vi "NI DOCO DEMO.vi"() -> ()   [LabVIEW 2018]
uses:
  <vilib>/DAQmx/write.llb/DAQmx Write (Digital Wfm 1Chan NSamp).vi
  <vilib>/DAQmx/write.llb/DAQmx Write (Analog Wfm 1Chan NSamp).vi
  <vilib>/DAQmx/create/channels.llb/DAQmx Create Channel (AO-Voltage-Basic).vi
  <vilib>/DAQmx/configure/timing.llb/DAQmx Timing (Sample Clock).vi
  <vilib>/DAQmx/create/channels.llb/DAQmx Create Channel (DO-Digital Output).vi
  <vilib>/Waveform/DWDTOps.llb/DWDT Boolean Array to Digital.vi
  <vilib>/Waveform/WDTOps.llb/WDT Append Waveforms DBL.vi
  <vilib>/DAQmx/miscellaneous.llb/DAQmx Fill In Error Info.vi
  <vilib>/Waveform/DWDTOps.llb/DWDT Uncompress Digital.vi
  <vilib>/Waveform/DWDTOps.llb/DWDT Append Digital Samples.vi
  <vilib>/measure/NI_MABase.lvlib
panel:
  out "Numeric":u32
  in  "Enum":enum16{"A A", "A B", "B B", "B A"}(ring)
  in  "stop 2":bool
  out "Mixed Signal Graph":T1(graph)
  in  "stop":bool
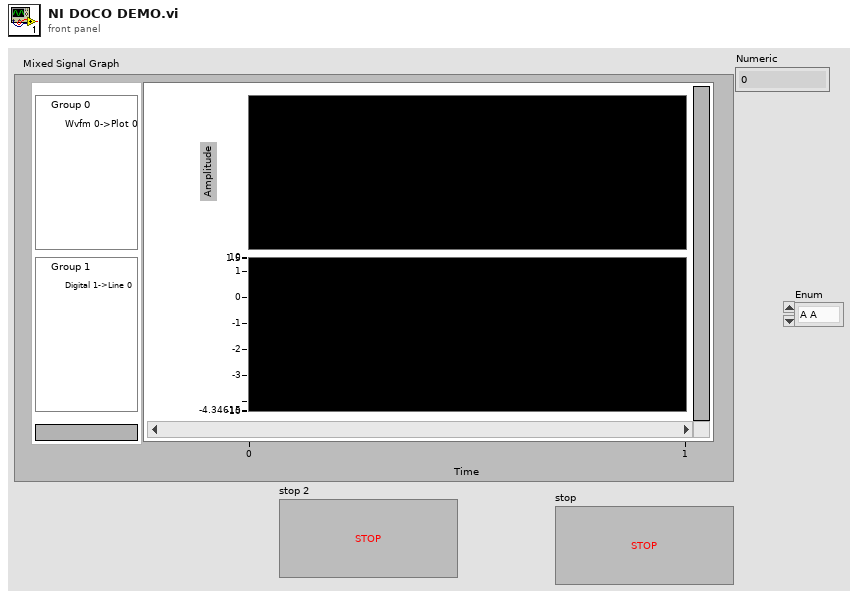
[diagram p1: front panel]
types:
  T1 = cluster{"signal out":waveform(dbl), "digital waveform":digitalwaveform}
  T2 = cluster{"waveform out":waveform(dbl), "output waveform":digitalwaveform}
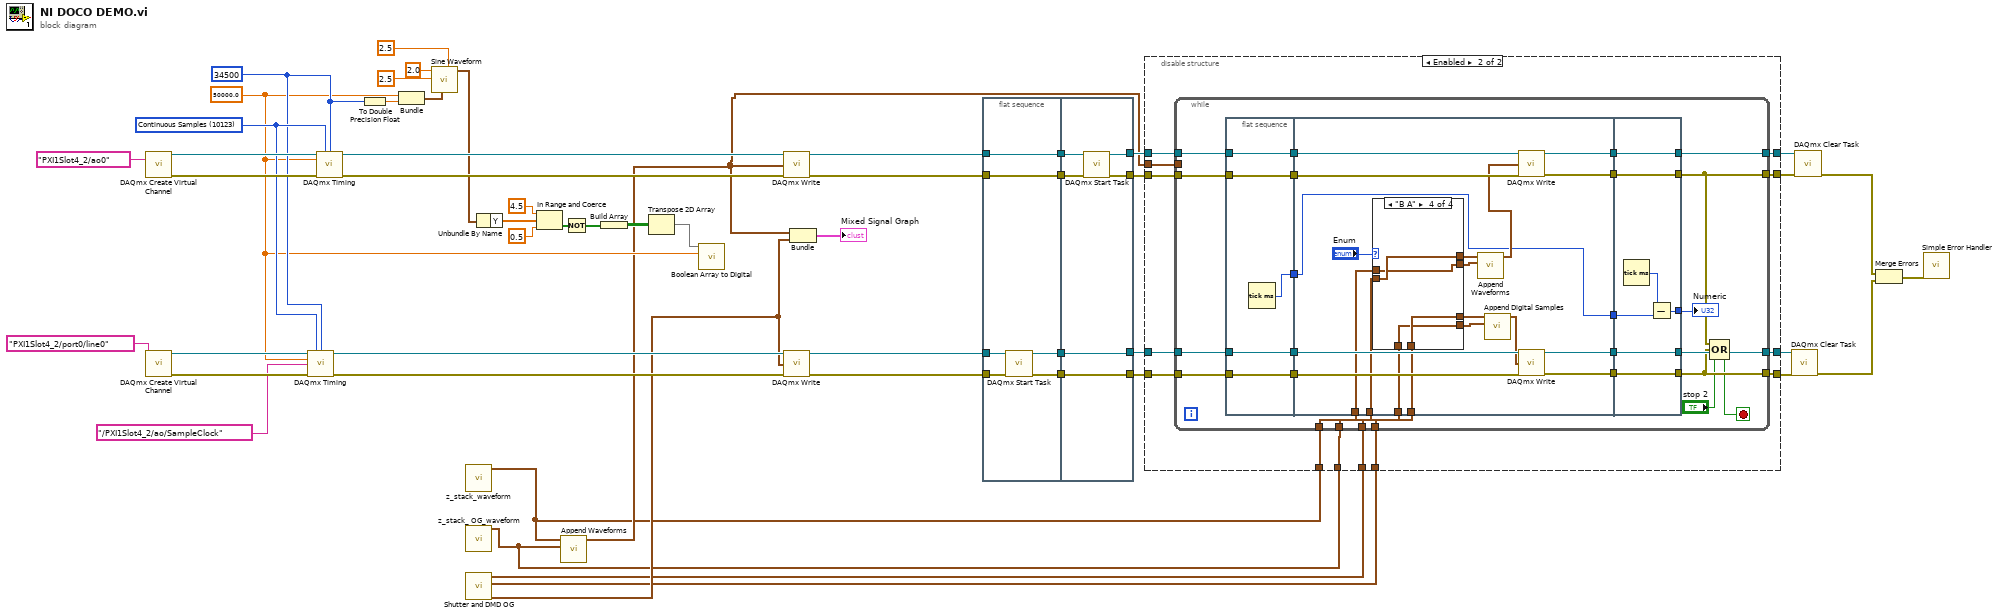
[diagram p0: block diagram]
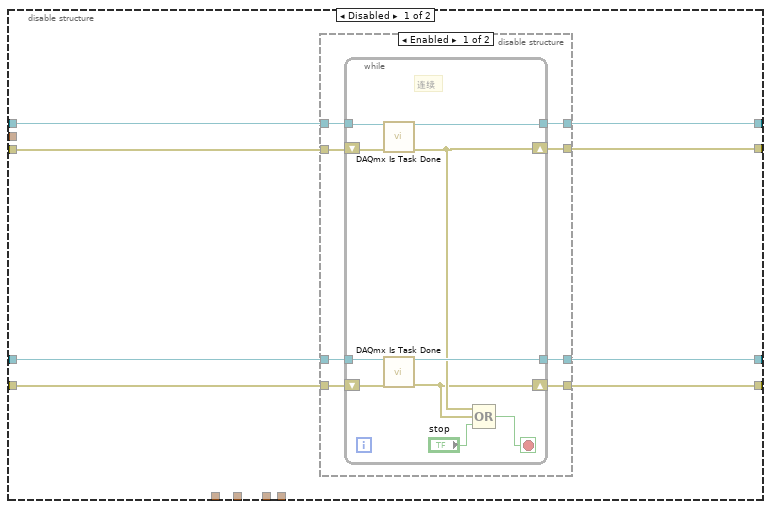
[diagram p2: hidden frame]
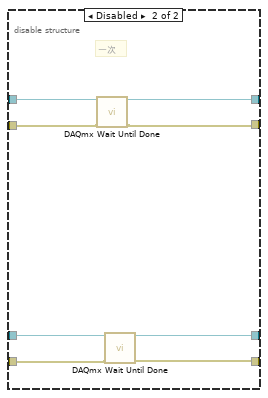
[diagram p3: hidden frame]
diagram:
  w42 = 34500 ("samples per channel")
  w47 = 10123 items=["Finite Samples"=10178, "Continuous Samples"=10123, "Hardware Timed Single Point"=12522] ("sample mode")
  w14 = 50000.0 ("rate")
  n1 = call-poly <vilib>:"DAQmx Create Virtual Channel.vi"("physical channels"=tag "PXI1Slot4_2/ao0") -> ("task out"=w52:refnum<k21>, "error out"=w51:errorcluster)  [unwired: 13 in]
  n2 = call-poly <vilib>:"DAQmx Create Virtual Channel.vi"("lines"=tag "PXI1Slot4_2/port0/line0") -> ("task out"=w48:refnum<k21>, "error out"=w49:errorcluster)  [unwired: 13 in]
  n3 = call-poly <vilib>:"DAQmx Timing.vi"("task/channels in"=w48, "sample mode"=w47, "samples per channel"=w42, "rate"=w14, "source"=tag "/PXI1Slot4_2/ao/SampleClock", "error in"=w49) -> ("task out"=w12:refnum<k21>, "error out"=w9:errorcluster)  [unwired: 8 in]
  n4 = call-poly <vilib>:"DAQmx Timing.vi"("task/channels in"=w52, "sample mode"=w47, "samples per channel"=w42, "rate"=w14, "error in"=w51) -> ("task out"=w45:refnum<k21>, "error out"=w44:errorcluster)  [unwired: 9 in]
  n5 = To Double Precision Float(number=w42) -> (double precision float=w43:dbl)
  n6 = Bundle("rate"=w14, w43) -> (w41:cluster{"rate":dbl, dbl})  [unwired: 1 in]
  n7 = call <vilib>:"Sine Waveform.vi"("offset"=2.5, "sampling info"=w41, "amplitude"=2.5, "frequency"=2.0) -> ("signal out"=w8:waveform(dbl))  [unwired: 6 in, 1 out]
  n8 = call "z_stack_waveform.vi"() -> ("waveform out"=w4:waveform(dbl))  [unwired: 9 in, 2 out]
  n9 = call "z_stack_ OG_waveform.vi"() -> ("waveform out"=w3:waveform(dbl))  [unwired: 15 in, 4 out]
  n10 = call "Shutter and DMD OG.vi"() -> ("output waveform"=w5:digitalwaveform, "output waveform 2"=w1:digitalwaveform, "output waveform1"=w2:digitalwaveform)  [unwired: 8 in]
  n11 = Unbundle By Name(w8) -> ("Y"=w20:dbl[])
  n12 = In Range and Coerce(upper limit=4.5 ("offset"), x=w20, lower limit=0.5 ("offset")) -> (In Range?=w17:bool[])  [unwired: 1 out]
  n13 = call-poly <vilib>:"Append Waveforms.vi"("waveform B"=w3, "waveform A"=w4) -> ("waveform out"=w6:waveform(dbl))  [unwired: 8 in, 1 out]
  n14 = Not(x=w17) -> (.not. x?=w16:bool[])
  n15 = Build Array(w16) -> (w15:bool[][])
  n16 = Transpose 2D Array(2D array=w15) -> (transposed array=w13:bool[][])
  n17 = call-poly <vilib>:"Boolean Array to Digital.vi"("sample rate"=w14, "boolean array"=w13) -> ()  [unwired: 8 in, 2 out]
  n18 = call-poly <vilib>:"DAQmx Write.vi"("task/channels in"=w45, "data"=w6, "error in"=w44) -> ("task out"=w37:refnum<k21>, "error out"=w33:errorcluster)  [unwired: 10 in, 1 out]
  n19 = call-poly <vilib>:"DAQmx Write.vi"("task/channels in"=w12, "data"=w5, "error in"=w9) -> ("task out"=w11:refnum<k21>, "error out"=w10:errorcluster)  [unwired: 10 in, 1 out]
  n20 = Bundle("waveform out"=w6, "output waveform"=w5) -> (→"Mixed Signal Graph":T2)  [unwired: 1 in]
  n21 = flat-sequence {
    tunnel: w37 -> [w59]
    tunnel: w11 -> [w58]
    tunnel: w10 -> [w57]
    tunnel: [w59] -> w36
    tunnel: [w56] -> w35
    tunnel: [w55] -> w34
    tunnel: w33 -> [w54]
    tunnel: [w54] -> w32
    tunnel: w36 -> [w63]
    tunnel: [w65] -> w29
    tunnel: w35 -> [w65]
    tunnel: [w64] -> w28
    tunnel: w34 -> [w64]
    tunnel: [w62] -> w31
    tunnel: w32 -> [w61]
    tunnel: [w60] -> w30
    frame #0 {
      n22 = call <vilib>:"DAQmx Start Task.vi"("task/channels in"=w58, "error in"=w57) -> ("task out"=w56:refnum<k21>, "error out"=w55:errorcluster)  [unwired: 12 in]
    }
    frame #1 {
      n23 = call <vilib>:"DAQmx Start Task.vi"("task/channels in"=w63, "error in"=w61) -> ("task out"=w62:refnum<k21>, "error out"=w60:errorcluster)  [unwired: 12 in]
    }
  }
  n24 = disable-structure shown="Enabled" {
    disable-tunnel: w31 -> [w73 w112]
    disable-tunnel: w30 -> [w72 w111]
    disable-tunnel: w29 -> [w71 w110]
    disable-tunnel: w28 -> [w70 w109]
    disable-tunnel: [w69 w107] -> w27
    disable-tunnel: [w68 w108] -> w26
    disable-tunnel: [w67 w106] -> w25
    disable-tunnel: [w66 w105] -> w24
    disable-tunnel: w6 -> [_ w104]
    disable-tunnel: w4 -> [_ w103]
    disable-tunnel: w3 -> [_ w102]
    disable-tunnel: w2 -> [_ w101]
    disable-tunnel: w1 -> [_ w100]
    frame Disabled {
      n25 = disable-structure shown="Enabled" {
        disable-tunnel: w73 -> [w81 w99]
        disable-tunnel: w72 -> [w80 w98]
        disable-tunnel: w71 -> [w79 w95]
        disable-tunnel: w70 -> [w78 w92]
        disable-tunnel: [w77 w96] -> w69
        disable-tunnel: [w76 w97] -> w68
        disable-tunnel: [w75 w94] -> w67
        disable-tunnel: [w74 w93] -> w66
        frame Enabled {
          n26 = while {
            tunnel: w81 -> [w91]
            tunnel: w79 -> [w89]
            tunnel: [w85] -> w75
            tunnel: [w84] -> w77
            shift-right: [w83] -> w76
            shift-left: w80 -> [w90]
            shift-right: [w82] -> w74
            shift-left: w78 -> [w88]
            stop <- w86 stop-if-true
            # "连续"
            n27 = call <vilib>:"DAQmx Is Task Done.vi"("task/channels in"=w91, "error in"=w90) -> ("task out"=w84:refnum<k21>, "error out"=w83:errorcluster)  [unwired: 11 in, 1 out]
            n28 = call <vilib>:"DAQmx Is Task Done.vi"("task/channels in"=w89, "error in"=w88) -> ("task out"=w85:refnum<k21>, "error out"=w82:errorcluster)  [unwired: 11 in, 1 out]
            n29 = Compound Arithmetic op=OR(w83, w82, "stop") -> (w86:bool)
          }
        }
        frame Disabled {
          # "一次"
          n30 = call <vilib>:"DAQmx Wait Until Done.vi"("task/channels in"=w99, "error in"=w98) -> ("task out"=w96:refnum<k21>, "error out"=w97:errorcluster)  [unwired: 12 in]
          n31 = call <vilib>:"DAQmx Wait Until Done.vi"("task/channels in"=w95, "error in"=w92) -> ("task out"=w94:refnum<k21>, "error out"=w93:errorcluster)  [unwired: 12 in]
        }
      }
    }
    frame Enabled {
      n32 = while {
        tunnel: w112 -> [w135]
        tunnel: w111 -> [w134]
        tunnel: w110 -> [w137]
        tunnel: w109 -> [w136]
        tunnel: [w131] -> w108
        tunnel: [w133] -> w107
        tunnel: [w132] -> w106
        tunnel: [w130] -> w105
        tunnel: w104 -> [_]
        tunnel: w103 -> [w127]
        tunnel: w102 -> [w126]
        tunnel: w101 -> [w125]
        tunnel: w100 -> [w124]
        stop <- w129 stop-if-true
        n33 = flat-sequence {
          tunnel: w134 -> [w139]
          tunnel: w135 -> [w140]
          tunnel: w136 -> [w141]
          tunnel: w137 -> [w142]
          tunnel: [w142] -> w123
          tunnel: [w141] -> w122
          tunnel: [w140] -> w121
          tunnel: [w139] -> w120
          tunnel: [w138] -> w115
          tunnel: w127 -> [w151]
          tunnel: w126 -> [w150]
          tunnel: w125 -> [w149]
          tunnel: w124 -> [w148]
          tunnel: w123 -> [w162]
          tunnel: w122 -> [w161]
          tunnel: w121 -> [w160]
          tunnel: w120 -> [w159]
          tunnel: [w158] -> w119
          tunnel: [w157] -> w118
          tunnel: [w156] -> w117
          tunnel: [w155] -> w116
          tunnel: w115 -> [w143]
          tunnel: [w143] -> w114
          tunnel: [w178] -> w130
          tunnel: [w179] -> w131
          tunnel: [w180] -> w132
          tunnel: [w181] -> w133
          tunnel: w119 -> [w181]
          tunnel: w118 -> [w180]
          tunnel: w117 -> [w179]
          tunnel: w116 -> [w178]
          tunnel: w114 -> [w176]
          tunnel: [w175] -> w113
          frame #0 {
            n34 = Tick Count (ms)() -> (millisecond timer value=w138:u32)
          }
          frame #1 {
            n35 = case shown="\"B A\"" "Enum" {
              tunnel: w151 -> [w164 w168 _ w173]
              tunnel: w150 -> [_ w167 w170 w174]
              tunnel: w149 -> [w163 w166 _ w171]
              tunnel: w148 -> [_ w165 w169 w172]
              tunnel: [w164 w168 w170 w174] -> w147
              tunnel: [w164 w167 w170 w173] -> w146
              tunnel: [w163 w166 w169 w172] -> w145
              tunnel: [w163 w165 w169 w171] -> w144
              frame "A A", Default {
              }
              frame "A B" {
              }
              frame "B B" {
              }
              frame "B A" {
              }
            }
            n36 = call-poly <vilib>:"Append Waveforms.vi"("waveform B"=w146, "waveform A"=w147) -> ("waveform out"=w153:waveform(dbl))  [unwired: 8 in, 1 out]
            n37 = call-poly <vilib>:"Append Digital Samples.vi"("digital waveform B"=w144, "digital waveform A"=w145) -> ("digital waveform out"=w152:digitalwaveform)  [unwired: 8 in, 1 out]
            n38 = call-poly <vilib>:"DAQmx Write.vi"("task/channels in"=w160, "data"=w153, "error in"=w159) -> ("task out"=w158:refnum<k21>, "error out"=w156:errorcluster)  [unwired: 10 in, 1 out]
            n39 = call-poly <vilib>:"DAQmx Write.vi"("task/channels in"=w162, "data"=w152, "error in"=w161) -> ("task out"=w157:refnum<k21>, "error out"=w155:errorcluster)  [unwired: 10 in, 1 out]
          }
          frame #2 {
            n40 = Tick Count (ms)() -> (millisecond timer value=w177:u32)
            n41 = Subtract(x=w177, y=w176) -> (x-y=w175:u32)
          }
        }
        n42 = Compound Arithmetic op=OR(w131, w130, "stop 2") -> (w129:bool)
        "Numeric" <- w113
      }
    }
  }
  n43 = call <vilib>:"DAQmx Clear Task.vi"("task in"=w25, "error in"=w24) -> ("error out"=w22:errorcluster)  [unwired: 13 in]
  n44 = call <vilib>:"DAQmx Clear Task.vi"("task in"=w27, "error in"=w26) -> ("error out"=w23:errorcluster)  [unwired: 13 in]
  n45 = Merge Errors(w23, w22) -> (w21:errorcluster)
  n46 = call <vilib>:"Simple Error Handler.vi"("error in (no error)"=w21) -> ()  [unwired: 4 in, 5 out]
